vi "Com Send and Responce.vi"(6 "Type":T3(ring), 7 "Aceptable Responce Array":string[](array[string]), 8 "Error":errorcluster, 9 "Read Times":T1, 10 "Command String":string, 11 "Com":refnum<visa-resource-name>) -> (0 "Error Out":errorcluster, 1 "Read Status Out":T2, 2 "Responce Out":string, 3 "Com Out":refnum<visa-resource-name>)   [LabVIEW 2020]
uses:
  TypeDefs_Utility/ENUM_Com_Read Status.ctl
  TypeDefs_Utility/Cluster_Com_Read Times.ctl
panel:
  # ":CARD:PICK?\\stesttwo,1,100\\n"
  # ":FILE:MEAS\\stest3\\n"
  # "INTE\\s1S\\n"
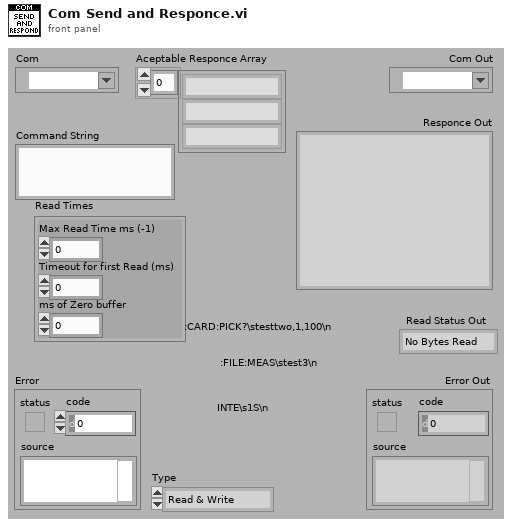
[diagram p1: front panel]
types:
  T1 = typedef "Cluster_Com_Read Times.ctl" = cluster{"Max Read Time ms (-1)":i32, "Timeout for first Read (ms)":u32, "ms of Zero buffer":u32}
  T2 = typedef "ENUM_Com_Read Status.ctl" = enum16{"No Bytes Read", "Bytes Read", "Stop String Read"}
  T3 = enum16{"Read & Write", "Read Only", "Write Only"}
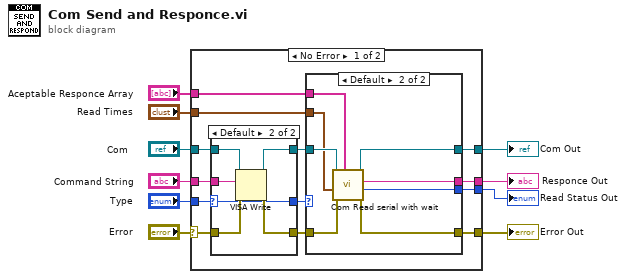
[diagram p0: block diagram]
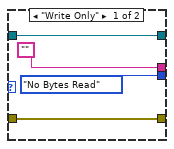
[diagram p2: hidden frame]
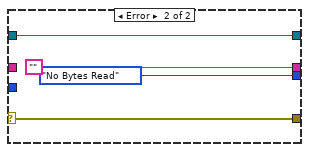
[diagram p4: hidden frame]
diagram:
  n1 = case shown="No Error" "Error" {
    selector: "Error" -> [w16 w48]
    tunnel: [w23 ""] -> w10
    tunnel: [w22 w48] -> w9
    tunnel: [w18 w47] -> w8
    tunnel: [w17 ENUM_Com_Read_Status."No Bytes Read" ("Status Out")] -> w7
    tunnel: "Com" -> [w19 w47]
    tunnel: "Type" -> [w13 _]
    tunnel: "Command String" -> [w15 _]
    tunnel: "Read Times" -> [w14 _]
    tunnel: "Aceptable Responce Array" -> [w11 _]
    frame No Error {
      n2 = case shown="Default" w13 {
        selector: w13 -> [w36 w39]
        tunnel: w15 -> [_ w44]
        tunnel: w16 -> [w38 w43]
        tunnel: [w38 w42] -> w21
        tunnel: [w37 w41] -> w20
        tunnel: w19 -> [w37 w40]
        tunnel: [w36 w39] -> w12
        frame "Read Only" {
        }
        frame Default {
          n3 = VISA Write(VISA resource name=w40, write buffer=w44, error in (no error)=w43) -> (VISA resource name out=w41:refnum<visa-resource-name>, error out=w42:errorcluster)  [unwired: 1 out]
        }
      }
      n4 = case shown="Default" w12 {
        tunnel: ["" w31] -> w23
        tunnel: [w27 w34] -> w22
        tunnel: w21 -> [w27 w35]
        tunnel: w20 -> [w25 w33]
        tunnel: [w25 w32] -> w18
        tunnel: [ENUM_Com_Read_Status."No Bytes Read" ("Responce Match Index\n-1 No Match From Last Read\n-2 No Responce Timeout\n-3 No Responce Last Read Out") w30] -> w17
        tunnel: w14 -> [_ w29]
        tunnel: w11 -> [_ w28]
        frame "Write Only" {
        }
        frame Default {
          n5 = call "Com Read serial with wait.vi"("Stop String array"=w28, "Error"=w35, "Read Times"=w29, "Com"=w33) -> ("Error Out"=w34:errorcluster, "Status Out"=w30:T2, "Read String Out"=w31:string, "Com Out"=w32:refnum<visa-resource-name>)  [unwired: 4 in]
        }
      }
    }
    frame Error {
    }
  }
  "Responce Out" <- w10
  "Error Out" <- w9
  "Com Out" <- w8
  "Read Status Out" <- w7
